vi "Display Units.vi"(8 "error in (no error)":errorcluster, 11 "VISA resource name":refnum<visa-resource-name>) -> (0 "error out":errorcluster, 2 "Units":string, 3 "VISA resource name out":refnum<visa-resource-name>)   [LabVIEW 2013, in "Newport 1830-C.lvlib"]
doc: "Reads units from instrument and ouputs symbol as a string."
uses:
  Newport 1830-C.lvlib
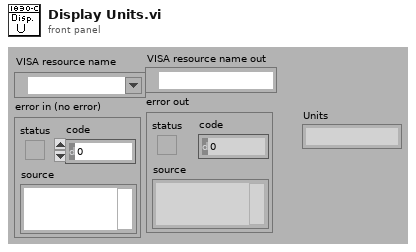
[diagram p1: front panel]
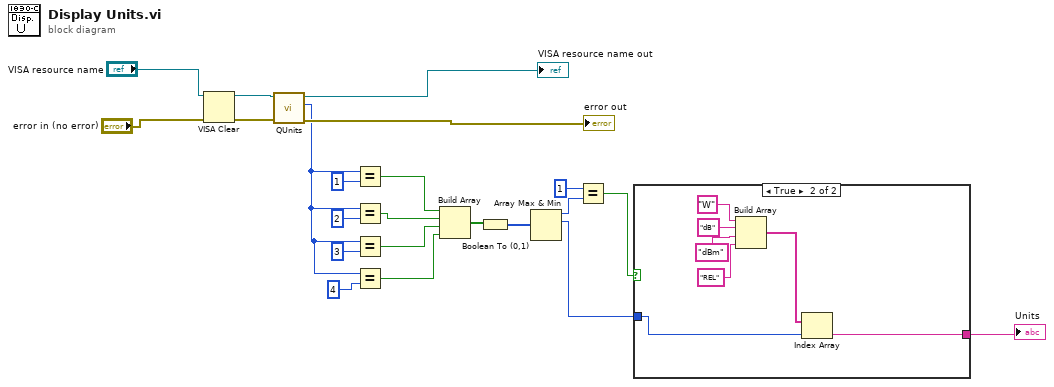
[diagram p0: block diagram]
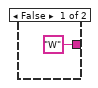
[diagram p2: hidden frame]
diagram:
  n1 = VISA Clear(VISA resource name="VISA resource name", error in (no error)="error in (no error)") -> (VISA resource name out=w1:refnum<visa-resource-name>, error out=w3:errorcluster)
  n2 = call "QUnits.vi"("error in (no error)"=w3, "VISA resource name"=w1) -> ("error out"=→"error out":errorcluster, "Units"=w20:u32, "VISA resource name out"=→"VISA resource name out":refnum<visa-resource-name>)  [unwired: 6 in, 1 out]
  n3 = Equal?(x=w20, y=1) -> (x = y?=w15:bool)
  n4 = Equal?(x=w20, y=2) -> (x = y?=w14:bool)
  n5 = Equal?(x=w20, y=3) -> (x = y?=w13:bool)
  n6 = Equal?(x=w20, y=4) -> (x = y?=w12:bool)
  n7 = Build Array(w15, w14, w13, w12) -> (w11:bool[])
  n8 = Boolean To (0,1)(Boolean=w11) -> (0, 1=w10:i16[])
  n9 = Array Max & Min(array=w10) -> (max value=w7:i16, max index (indices)=w9:i32)  [unwired: 2 out]
  n10 = Equal?(x=i16 1, y=w7) -> (x = y?=w5:bool)
  n11 = case shown="True" w5 {
    tunnel: w9 -> [_ w25]
    tunnel: ["W" w24] -> w8
    frame False {
    }
    frame True {
      n12 = Build Array("W", "dB", "dBm", "REL") -> (w26:string[])
      n13 = Index Array(array=w26, index=w25) -> (element=w24:string)
    }
  }
  "Units" <- w8
